vi "intakeLoop.vi"   [LabVIEW 2017]
uses:
  <vilib>/Rock Robotics/WPI/Solenoid/WPI_SolenoidValue.ctl
  <vilib>/Platform/TimedLoop/XDataNode/timing_clust.ctl
  <vilib>/Platform/TimedLoop/XDataNode/nitl_modes.ctl
  <vilib>/Platform/TimedLoop/XDataNode/wakeup.ctl
  <vilib>/Rock Robotics/WPI/Solenoid/WPI_SolenoidGetEnum.vi
  <vilib>/Rock Robotics/WPI/Solenoid/WPI_SolenoidSetEnum.vi
  <vilib>/platform/TimedLoop/XDataNode/XDataNode.xnode
  <vilib>/Platform/TimedLoop/XDataNode/XDNodeRunTimeDep.lvlib
types:
  T1 = typedef "WPI_SolenoidValue.ctl" = enum16{"Off", "On", "Forward", "Reverse"}
  T2 = typedef "WPI_SolenoidDevRef.ctl" = cluster{"DevStatus":errorcluster, "Pneumatics Control Module":u8, "Forward Solenoid Channel":T3, "Reverse Solenoid Channel":T3}
  T3 = typedef "WPI_SolenoidChannel.ctl" = enum8{"Solenoid 0", "Solenoid 1", "Solenoid 2", "Solenoid 3", "Solenoid 4", "Solenoid 5", "Solenoid 6", "Solenoid 7", "Invalid"}
  T4 = typedef "XDNodeRunTimeDep.lvlib/timing_clust.ctl" = cluster{"Expected End [f-1]":u64, "Actual End [f-1]":u64, "Finished Late? [f-1]":bool, "Expected End [i-1]":u64, "Actual End [i-1]":u64, "Finished Late? [i-1]":bool, "Expected Start [i]":u64, "Actual Start [i]":u64, "Expected Start [f]":u64, "Actual Start [f]":u64, "Source Name":string, "Structure Name":string, "Period":i64, "Deadline":i64, "Offset":i64, "Start":i64, "Priority":i32, "Timeout":i32, "Mode":T5, "Wakeup Reason":T6, "Error":errorcluster, "Source Type":string, "Secondary Source Type":string, "Global End Time":u64, "Global Start Time":u64, "Frame Duration":u64, "Iteration Duration":u64, "Assigned CPU":i32, "I/O Scan Engine Mode":u32}
  T5 = typedef "XDNodeRunTimeDep.lvlib/nitl_modes.ctl" = enum32{"No Change", "Process missed periods, maintain original phase", "Discard missed periods, maintain original phase", "Process missed periods, ignore original phase", "Discard missed periods, ignore original phase"}
  T6 = typedef "XDNodeRunTimeDep.lvlib/wakeup.ctl" = enum32{"Normal", "Aborted", "Asynchronous wakeup", "Timing source error", "Timed loop error", "Timeout"}
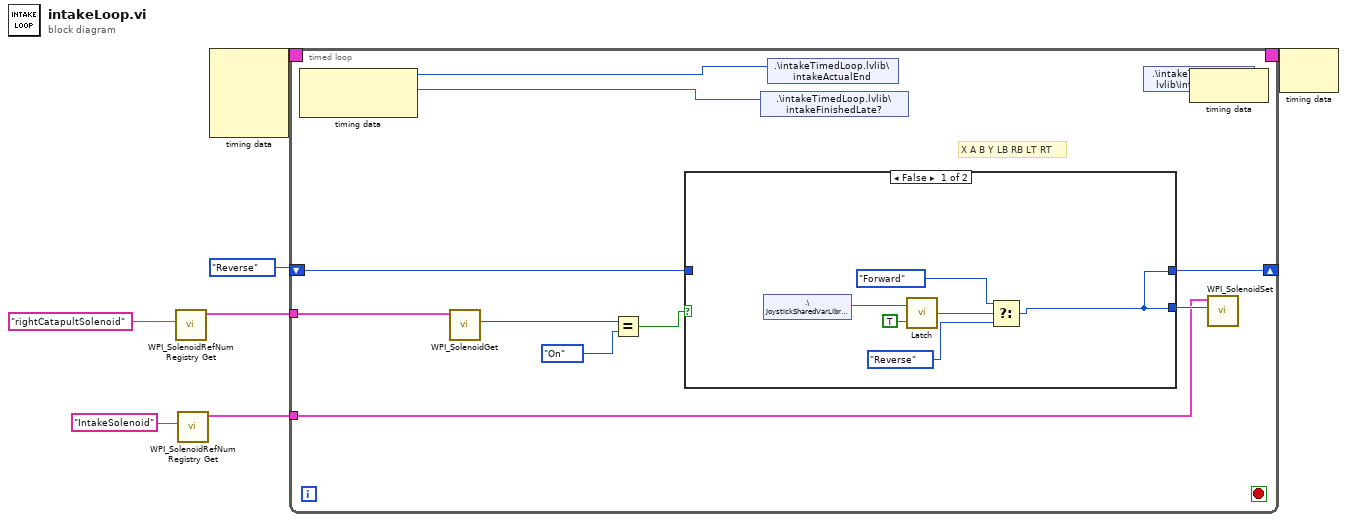
[diagram p0: block diagram]
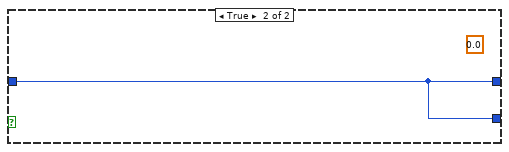
[diagram p2: hidden frame]
diagram:
  n1 = call <vilib>:"WPI_SolenoidRefNum Registry Get.vi"("refnum name"="rightCatapultSolenoid") -> ("SolenoidDevRef"=w1:T2)  [unwired: 9 in, 1 out]
  n2 = call <vilib>:"WPI_SolenoidRefNum Registry Get.vi"("refnum name"="IntakeSolenoid") -> ("SolenoidDevRef"=w3:T2)  [unwired: 9 in, 1 out]
  n3 = node-c288() -> (w7:T4)  [unwired: 4 in]
  n4 = timed-loop {
    timing: w7 -> [_]
    timing-out: [_] -> w6
    tunnel: w3 -> [w14]
    shift-right: [w13] -> _
    shift-left: WPI_SolenoidValue."Reverse" ("Value") -> [w10]
    tunnel: w1 -> [w8]
    stop <- _ stop-if-true
    # "X A B Y LB RB LT RT"
    n5 = node-c288() -> (w17:i64, w16:bool)  [unwired: 1 in]
    n6 = call-poly <vilib>:"WPI_SolenoidGet.vi"("SolenoidDevRef"=w8) -> ("Value"=w9:T1)  [unwired: 8 in, 2 out]
    n7 = Equal?(x=w9, y=WPI_SolenoidValue."On" ("Value")) -> (x = y?=w11:bool)
    n8 = case shown="False" w11 {
      tunnel: [w22 w25] -> w15
      tunnel: [w22 w25] -> w13
      tunnel: w10 -> [_ w25]
      frame False {
        n9 = shared-variable ".\\JoystickSharedVarLibrary.lvlib\\bButton"() -> (w24:bool)  [unwired: 1 in, 1 out]
        n10 = call <userlib>:"Latch.vi"("Edge"=TRUE, "In"=w24) -> ("Out"=w19:bool)
        n11 = Select(t=WPI_SolenoidValue."Forward" ("Value"), s=w19, f=WPI_SolenoidValue."Reverse" ("Value")) -> (s? t:f=w22:T1)
      }
      frame True {
        (unwired) 0.0 ("Output")
      }
    }
    n12 = shared-variable ".\\intakeTimedLoop.lvlib\\intakeFinishedLate?"(w16) -> ()  [unwired: 1 in, 1 out]
    n13 = shared-variable ".\\intakeTimedLoop.lvlib\\intakeActualEnd"(w17) -> ()  [unwired: 1 in, 1 out]
    n14 = shared-variable ".\\intakeTimedLoop.lvlib\\intakePeriod"() -> (w18:i64)  [unwired: 1 in, 1 out]
    n15 = node-c288(w18) -> ()  [unwired: 1 out]
    n16 = call-poly <vilib>:"WPI_SolenoidSet.vi"("Value"=w15, "SolenoidDevRef"=w14) -> ()  [unwired: 8 in, 2 out]
  }
  n17 = node-c288(w6) -> ()  [unwired: 1 out]
